vi "Test_TerminalReference_LatchingBoolean_Error.vi"(8 "error in (no error)":errorcluster, 11 "TestCase in":refnum<class "TestTransport.lvclass">) -> (0 "error out":errorcluster, 3 "TestCase out":refnum<class "TestTransport.lvclass">)   [LabVIEW 2017, in "TestTransport.lvclass"]
uses:
  TestTransport.lvclass
  TerminalReferenceBinding/TerminalReferenceBinding.lvclass
panel:
  in  "A Latching Button":bool
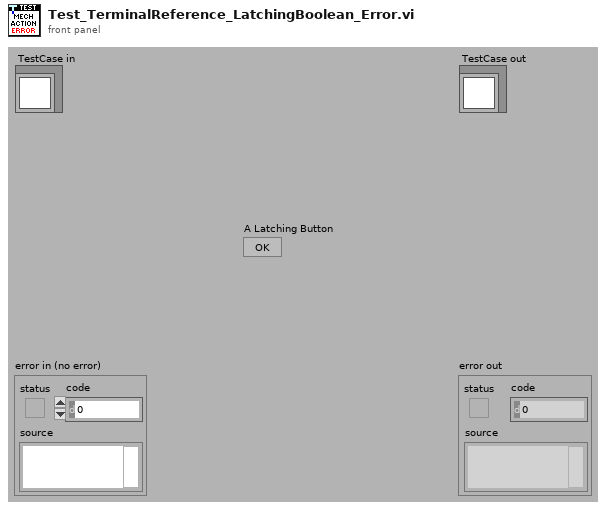
[diagram p1: front panel]
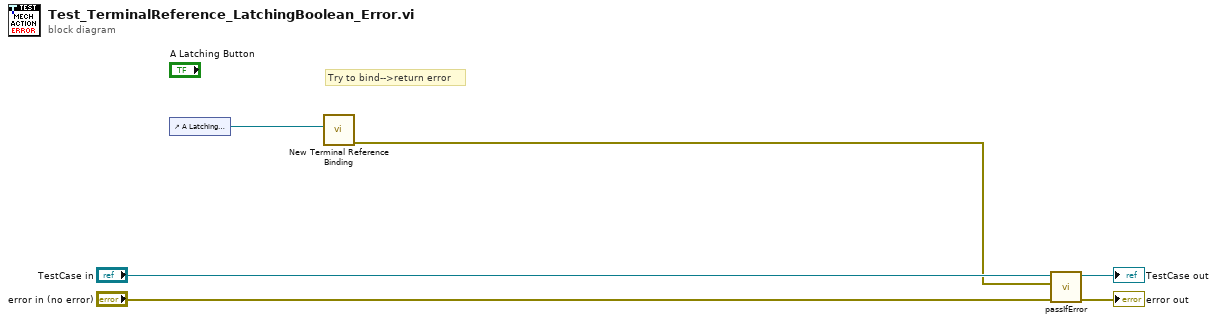
[diagram p0: block diagram]
diagram:
  # "Try to bind-->return error"
  n1 = control-ref of="A Latching Button"() -> (w3:refnum<vi>)
  n2 = call "New Terminal Reference Binding.vi"("Ctl Refnum"=w3) -> ("error out"=w2:errorcluster)  [unwired: 9 in, 1 out]
  n3 = call-dynamic "passIfError.vi"("error in (no error)"="error in (no error)", "error"=w2, "TestCase in"="TestCase in") -> ("error out"=→"error out":errorcluster, "TestCase out"=→"TestCase out":refnum<class "TestTransport.lvclass">)  [unwired: 7 in]
